vi "computer.vi"(0 "sen":dbl, 5 "off":dbl, 7 "range":i32, 9 "trig":sgl, 11 "错误输入（无错误）":errorcluster) -> (6 "结果":dbl, 15 "错误输出":errorcluster)   [LabVIEW 2009]
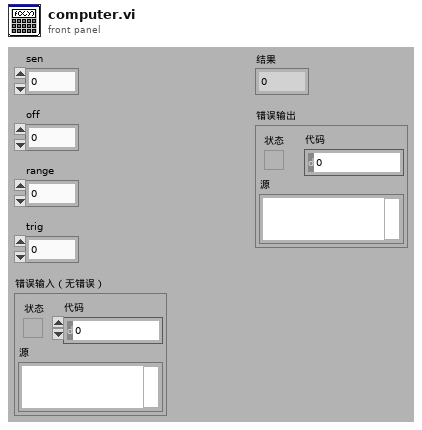
[diagram p1: front panel]
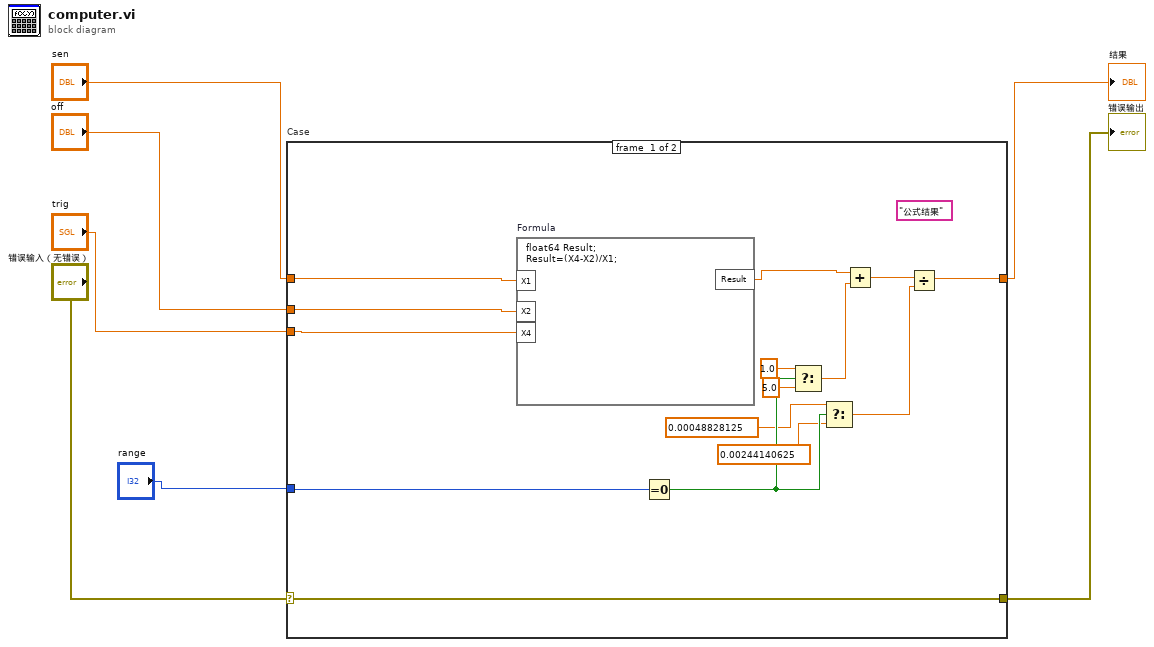
[diagram p0: block diagram]
diagram:
  n1 = case "Case" shown="无错误" "错误输入（无错误）" {
    selector: "错误输入（无错误）" -> [w19 w23]
    tunnel: [w16 _] -> w2
    tunnel: [w19 w23] -> w1
    tunnel: "sen" -> [w22 _]
    tunnel: "off" -> [w21 _]
    tunnel: "range" -> [w15 _]
    tunnel: "trig" -> [w20 _]
    frame #0 {
      (unwired) "公式结果" ("Name Modifier")
      n2 = formula code="float64 Result;\nResult=(X4-X2)/X1;"("X1"=w22, "X2"=w21, "X4"=w20) -> ("Result"=w17:dbl)
      n3 = Equal To 0?(x=w15) -> (x = 0?=w12:bool)
      n4 = Select(t=1.0, s=w12, f=5.0) -> (s? t:f=w14:dbl)
      n5 = Select(t=0.00048828125, s=w12, f=0.00244140625) -> (s? t:f=w13:dbl)
      n6 = Add(x=w17, y=w14) -> (x+y=w18:dbl)
      n7 = Divide(x=w18, y=w13) -> (x/y=w16:dbl)
    }
    frame #1 {
    }
  }
  "结果" <- w2
  "错误输出" <- w1
